vi "Temperature Control.vi"() -> ()   [LabVIEW 2014]
panel:
  in  "Board Type (Uno)":T1
  in  "COM Port":refnum<visa-resource-name>
  out "COLD":bool
  out "MODERATE":bool
  out "HOT":bool
  out "Thermometer":dbl(slide) scale=0.0..100.0
  out "Temprature Chart":dbl(graph)
  in  "Maximum":dbl(slide) scale=0.0..100.0 scale format="%^#_6g"
  in  "Minimum":dbl(slide) scale=0.0..100.0 scale format="%^#_5g"
  in  "Analog Channel":u8
  in  "?":bool
  # "TEMPERATURE CONTROL UNIT"
  # "VATSAL SHAH\nINDUS UNIVERSITY"
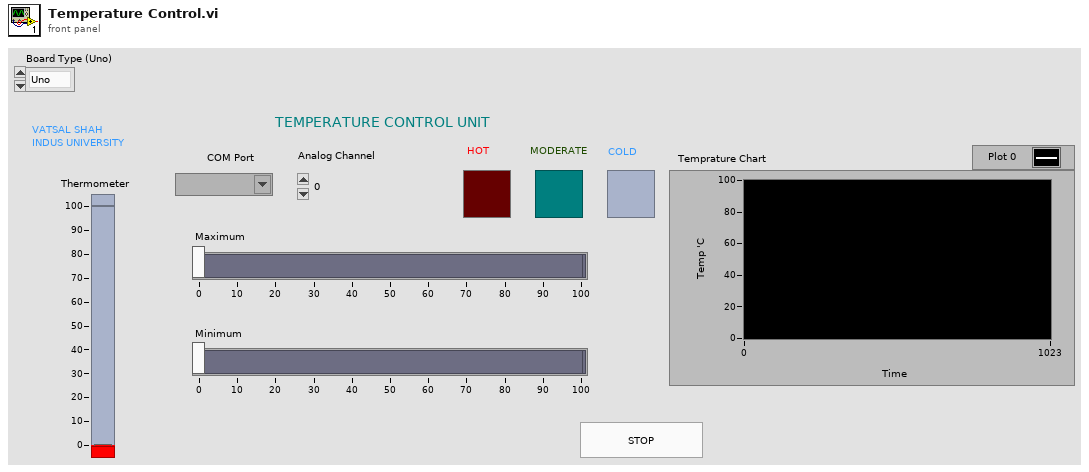
[diagram p1: front panel]
types:
  T1 = typedef "LabVIEW Interface for Arduino.lvlib/Board Type.ctl" = enum16{"Uno", "Dimuelanove w/Atmega 328", "Mega 2560"}
  T2 = typedef "LabVIEW Interface for Arduino.lvlib/Arduino Resource.ctl" = cluster{"VISA resource":refnum<visa-resource-name>, "Board Type":T1, "Connection Type":enum8{"USB / Serial"}, "Bytes Per Packet (15)":u8}
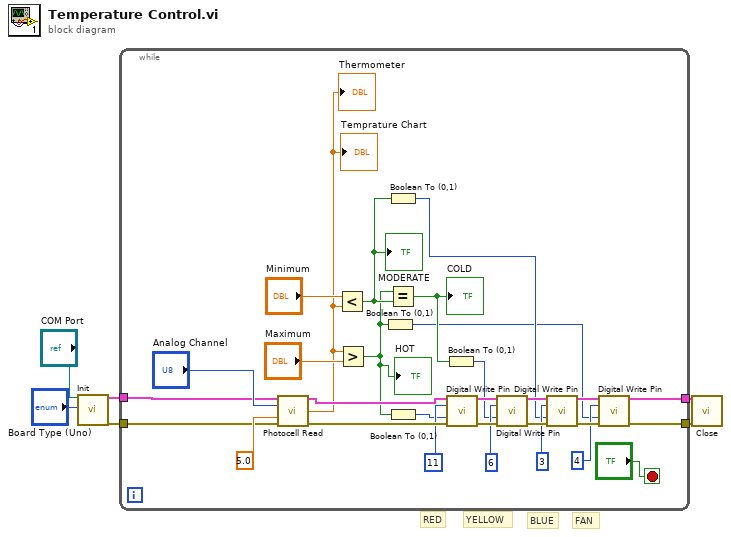
[diagram p0: block diagram]
diagram:
  # "FAN"
  # "BLUE"
  # "YELLOW"
  # "RED"
  n1 = call <vilib>:"Init.vi"("VISA resource"="COM Port", "Board Type (Uno)"="Board Type (Uno)") -> ("Arduino Resource"=w6:T2, "error out"=w4:errorcluster)  [unwired: 16 in]
  n2 = while {
    tunnel: w6 -> [w30]
    tunnel: [w26] -> w5
    tunnel: w4 -> [w25]
    tunnel: [w20] -> w3
    stop <- "?" stop-if-true
    n3 = call <vilib>:"Photocell Read.vi"("Arduino Resource"=w30, "Photo Cell Pin (0)"="Analog Channel", "Vcc (5)"=5.0, "error in"=w25) -> ("Arduino Resource"=w10:T2, "Light Intensity (0 - 100)"=w9:dbl, "error out"=w24:errorcluster)  [unwired: 9 in]
    "Thermometer" <- w9
    "Temprature Chart" <- w9
    n4 = Less?(x="Minimum", y=w9) -> (x < y?=w12:bool)
    "MODERATE" <- w12
    n5 = Greater?(x=w9, y="Maximum") -> (0:w8:bool)
    "HOT" <- w8
    n6 = Boolean To (0,1)(Boolean=w8) -> (0, 1=w7:i16)
    n7 = Boolean To (0,1)(Boolean=w12) -> (0, 1=w13:i16)
    n8 = Equal?(x=w8, y=w12) -> (x = y?=w11:bool)
    "COLD" <- w11
    n9 = Boolean To (0,1)(Boolean=w8) -> (0, 1=w15:i16)
    n10 = Boolean To (0,1)(Boolean=w11) -> (0, 1=w14:i16)
    n11 = call <vilib>:"Digital Write Pin.vi"("Arduino Resource"=w10, "Digital I/O Pin (0)"=u8 11, "Value (0)"=w15, "error in"=w24) -> ("Arduino Resource"=w29:T2, "error out"=w23:errorcluster)  [unwired: 10 in]
    n12 = call <vilib>:"Digital Write Pin.vi"("Arduino Resource"=w29, "Digital I/O Pin (0)"=u8 6, "Value (0)"=w14, "error in"=w23) -> ("Arduino Resource"=w28:T2, "error out"=w22:errorcluster)  [unwired: 10 in]
    n13 = call <vilib>:"Digital Write Pin.vi"("Arduino Resource"=w28, "Digital I/O Pin (0)"=u8 3, "Value (0)"=w13, "error in"=w22) -> ("Arduino Resource"=w27:T2, "error out"=w21:errorcluster)  [unwired: 10 in]
    n14 = call <vilib>:"Digital Write Pin.vi"("Arduino Resource"=w27, "Digital I/O Pin (0)"=u8 4, "Value (0)"=w7, "error in"=w21) -> ("Arduino Resource"=w26:T2, "error out"=w20:errorcluster)  [unwired: 10 in]
  }
  n15 = call <vilib>:"Close.vi"("Arduino Resource"=w5, "error in"=w3) -> ()  [unwired: 13 in, 1 out]
